vi "Culab Not Complex Graph.vi"(7 "nb_loop":i32=5, 8 "error in (no error)":errorcluster, 9 "C":refnum<class "T0D_SGL.lvclass">, 10 "B":refnum<class "T1D_SGL.lvclass">, 11 "A":refnum<class "T1D_SGL.lvclass">) -> (0 "error out":errorcluster, 3 "Dest out":refnum<class "T0D_SGL.lvclass">)   [LabVIEW 2020]
uses:
  <vilib>/Ngene/CuLab - GPU Accelerated Toolkit/Toolkit/Low_Level/Tensor_Classes/T_Children/T1D/T1D_Children/T1D_SGL/T1D_SGL.lvclass
  C:/Program Files/National Instruments/LabVIEW 2020/vi.lib/Ngene/CuLab - GPU Accelerated Toolkit/Toolkit/Low_Level/Tensor_Classes/Tensor.lvclass
  <vilib>/Ngene/CuLab - GPU Accelerated Toolkit/Toolkit/Low_Level/Tensor_Classes/T_Children/T0D/T0D_Children/T0D_SGL/T0D_SGL.lvclass
  <vilib>/Ngene/CuLab - GPU Accelerated Toolkit/Toolkit/API/Numeric/Add/T1D/CU_AddC_T1D_SGL.vi
  <vilib>/Ngene/CuLab - GPU Accelerated Toolkit/Toolkit/API/Numeric/Negate/T1D/CU_Negate_T1D_SGL.vi
  <vilib>/Ngene/CuLab - GPU Accelerated Toolkit/Toolkit/API/Numeric/Multiply/T1D/CU_Multiply_T1D_SGL.vi
  <vilib>/Ngene/CuLab - GPU Accelerated Toolkit/Toolkit/API/Numeric/Divide/T1D/CU_Divide_T1D_SGL.vi
  <vilib>/Ngene/CuLab - GPU Accelerated Toolkit/Toolkit/API/Numeric/Add Array Elements/T1D/CU_Add_Array_Elements_T1D_SGL.vi
  <vilib>/Ngene/CuLab - GPU Accelerated Toolkit/Toolkit/CuLab.lvlib
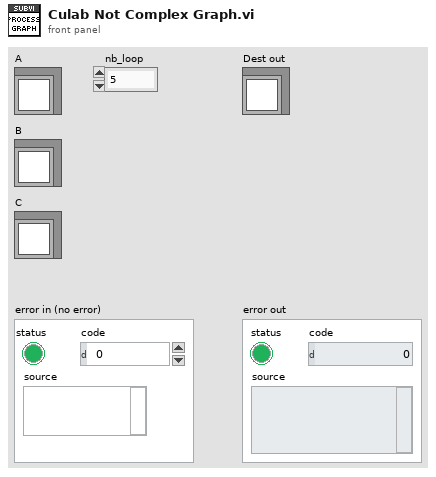
[diagram p1: front panel]
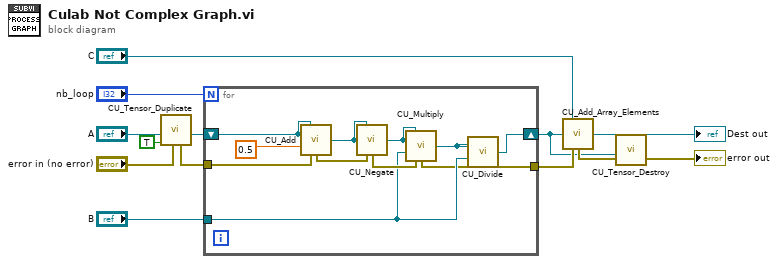
[diagram p0: block diagram]
diagram:
  n1 = call <vilib>:"CU_Tensor_Duplicate.vi"("error in (no error)"="error in (no error)", "Copy Data?"=TRUE, "Tensor in"="A") -> ("Duplicate out"=w11:refnum<class "T1D_SGL.lvclass">, "error out"=w5:errorcluster)  [unwired: 7 in]
  n2 = for {
    N: "nb_loop" -> [_]
    tunnel: "B" -> [w20]
    shift-right: [w19] -> w1
    shift-left: w11 -> [w22]
    tunnel: w5 -> [w24]
    tunnel: [w16] -> w4
    n3 = call-poly <vilib>:"CU_Add.vi"("Dest in"=w22, "x"=w22, "y"=sgl 0.5, "error in (no error)"=w24) -> ("Dest out"=w15:refnum<class "T1D_SGL.lvclass">, "error out"=w14:errorcluster)  [unwired: 10 in]
    n4 = call-poly <vilib>:"CU_Negate.vi"("Dest in"=w15, "x"=w15, "error in (no error)"=w14) -> ("Dest out"=w21:refnum<class "T1D_SGL.lvclass">, "error out"=w25:errorcluster)  [unwired: 11 in]
    n5 = call-poly <vilib>:"CU_Multiply.vi"("Dest in"=w21, "x"=w21, "y"=w20, "error in (no error)"=w25) -> ("Dest out"=w18:refnum<class "T1D_SGL.lvclass">, "error out"=w17:errorcluster)  [unwired: 10 in]
    n6 = call-poly <vilib>:"CU_Divide.vi"("Dest in"=w18, "x"=w18, "y"=w20, "error in (no error)"=w17) -> ("Dest out"=w19:refnum<class "T1D_SGL.lvclass">, "error out"=w16:errorcluster)  [unwired: 10 in]
  }
  n7 = call-poly <vilib>:"CU_Add_Array_Elements.vi"("Dest in"="C", "x"=w1, "error in (no error)"=w4) -> ("Dest out"=→"Dest out":refnum<class "T0D_SGL.lvclass">, "error out"=w8:errorcluster)  [unwired: 11 in]
  n8 = call <vilib>:"CU_Tensor_Destroy.vi"("error in (no error)"=w8, "Tensor in"=w1) -> ("error out"=→"error out":errorcluster)  [unwired: 9 in]
